vi "Flatten Value.vi"(8 "Error In":errorcluster, 11 "Int Array In":refnum<class "1D Int.lvclass">) -> (0 "Error Out":errorcluster, 1 "Value":string, 3 "Int Array Out":refnum<class "1D Int.lvclass">)   [LabVIEW 2017, in "Tree API.lvlib" / "1D Int.lvclass"]
uses:
  1D Int.lvclass
  Tree Manager/Tree.lvclass
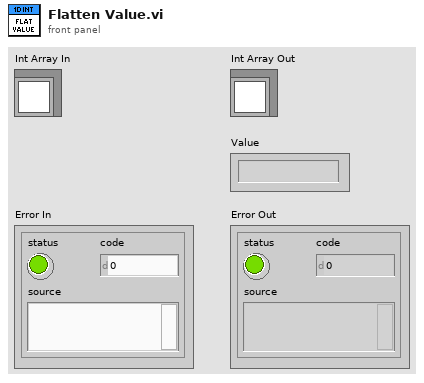
[diagram p1: front panel]
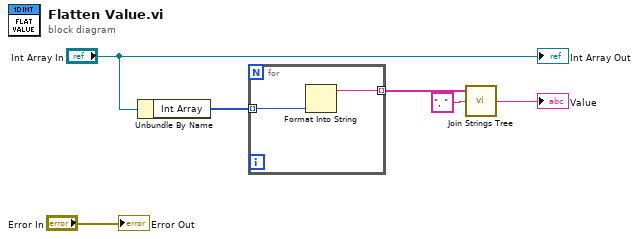
[diagram p0: block diagram]
diagram:
  n1 = Unbundle By Name("Int Array In") -> ("Int Array"=w6:i64[])
  n2 = for {
    tunnel: w6 -> [w8] mode=indexing
    tunnel: [w7] -> w5 mode=indexing
    n3 = Format Into String(w8) -> (resulting string=w7:string)  [unwired: 3 in, 1 out]
  }
  n4 = call "Join Strings Tree.vi"("Separator (,)"=", ", "Strings In"=w5) -> ("String"=→"Value":string)  [unwired: 1 in]
  "Int Array Out" <- "Int Array In"
  "Error Out" <- "Error In"
